vi "ADC.vi"() -> ()   [LabVIEW 2013]
panel:
  in  "ADC Rate":i32
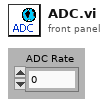
[diagram p1: front panel]
diagram:
